vi "Generate Timestamped Filepath.vi"(8 "Error In":errorcluster, 10 "appended filename":string) -> (0 "Error Out":errorcluster, 3 "timestamped relative filepath":path)   [LabVIEW 2020]
doc: "Generates a timestamped filepath with an appended user-specified name and the same directory containing the project."
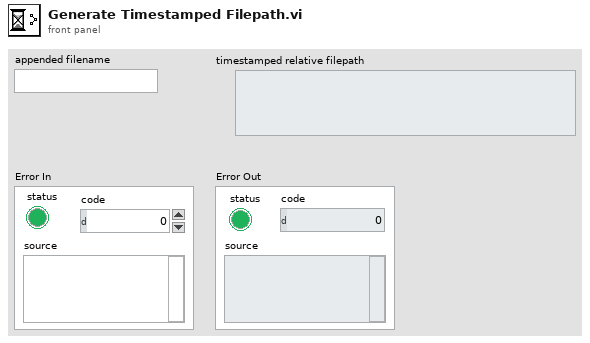
[diagram p1: front panel]
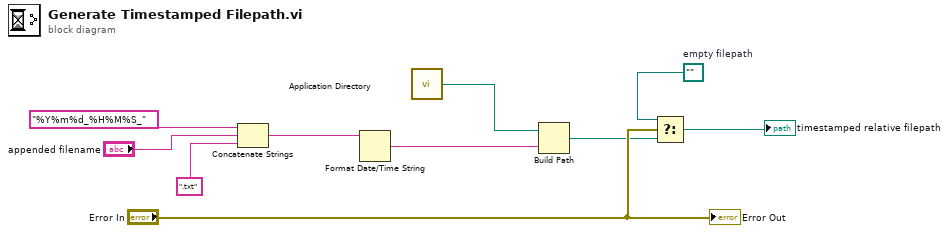
[diagram p0: block diagram]
diagram:
  w2 = path ""  # empty filepath
  n1 = Concatenate Strings "Concatenate Strings"("%Y%m%d_%H%M%S_" ("string"), "appended filename", ".txt" ("string")) -> (w8:string)
  n2 = Format Date/Time String(time format string (%c)=w8) -> (date/time string=w9:string)  [unwired: 2 in]
  n3 = call <vilib>:"Application Directory.vi"() -> ("Application Directory"=w10:path)
  n4 = Build Path(base path=w10, name or relative path=w9) -> (appended path=w3:path)
  n5 = Select(t=w2, s="Error In", f=w3) -> (s? t:f=→"timestamped relative filepath":path)
  "Error Out" <- "Error In"
